vi "niRFUtil MEAS Estimate IQ Imbalances.vi"(8 "Reference Waveform":T2 {"y" format="%.2f"; "dx" format="%^.2e"; "x0" format="%^.2e"}, 10 "Measured Waveform":T2 {"y" format="%.2f"; "dx" format="%^.2e"; "x0" format="%^.2e"}) -> (0 "Phase Imbalance (rad)":sgl, 1 "Gain Imbalance g (lin)":sgl, 2 "Channel Phase Offset (rad)":sgl, 3 "Normalization Factor (lin)":sgl, 4 "Imbalance Matrix":T1)   [LabVIEW 2015, in "niRFUtil.lvlib"]
doc: "<b>Joint Estmator for IQ gain and phase imbalance and channel gain and phase</b>\n\nThe VI estimates the IQ gain and phase imbalances together with channel gain and phase. In presence of IQ imbalances, these parameters depend on each other and need a joint estimation. \n\nAssumptions:\n1. Arbitrary complex time-domain baseband signal and corresponding complex time-domain baseband reference signal\n2. Frequency offset free input signal\n3. Arbitrary gain scaling of input signal\n4. Origin Offset free input signal \n\nThe estimation algorithm is documented in \n//RfProtocols/Kraken/niCDMA2k/dev/2.0/group/NID_Documents/General/IqImbalanceEstimation/IqImbalanceEstimation.pdf \n\nThe model used for definition of gain and phase imbalance is taken from:\nA. Georgiadis, \"Gain, phase imbalance, and phase noise effects on error vector magnitude,\" in IEEE Transactions on Vehicular Technology, vol. 53, no. 2, pp. 443-449, March 2004."
uses:
  niRFUtil.lvlib
  Includes/niRFUtil INC Complex Waveform.ctl
  Includes/niRFUtil INC Complex Array.ctl
  <vilib>/Analysis/Matrix/Datatypes/RealMatrix.ctl
  <vilib>/Analysis/Matrix/Numeric/Conversions/Array To Matrix - RA2.vi
  <vilib>/Analysis/Matrix/NI_Matrix.lvlib
panel:
  out "phaseChannelRef":dbl
  out "phaseImbalanceRef":dbl
  out "Gain ImbalanceRef (log)":dbl
  out "ChannelGain":dbl
  out "Gain ImbalanceRef (lin)":dbl
  out "phaseChannelRefDeg":dbl
  out "phaseImbalanceRefDeg":dbl
  out "Gain Imbalance g (dB)":sgl
  out "Channel Phase Offset (deg)":sgl
  out "Phase Imbalance (deg)":sgl
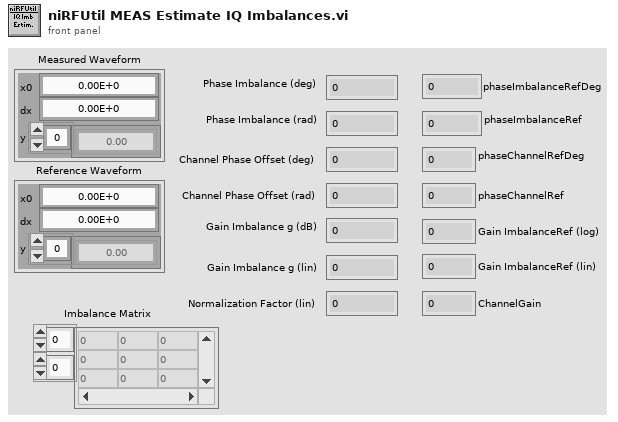
[diagram p1: front panel]
types:
  T1 = typedef "NI_Matrix.lvlib/RealMatrix.ctl" = dbl[][]
  T2 = typedef "niRFUtil.lvlib/niRFUtil INC Complex Waveform.ctl" = cluster{"x0":dbl, "dx":dbl, "y":T3}
  T3 = typedef "niRFUtil.lvlib/niRFUtil INC Complex Array.ctl" = csg[]
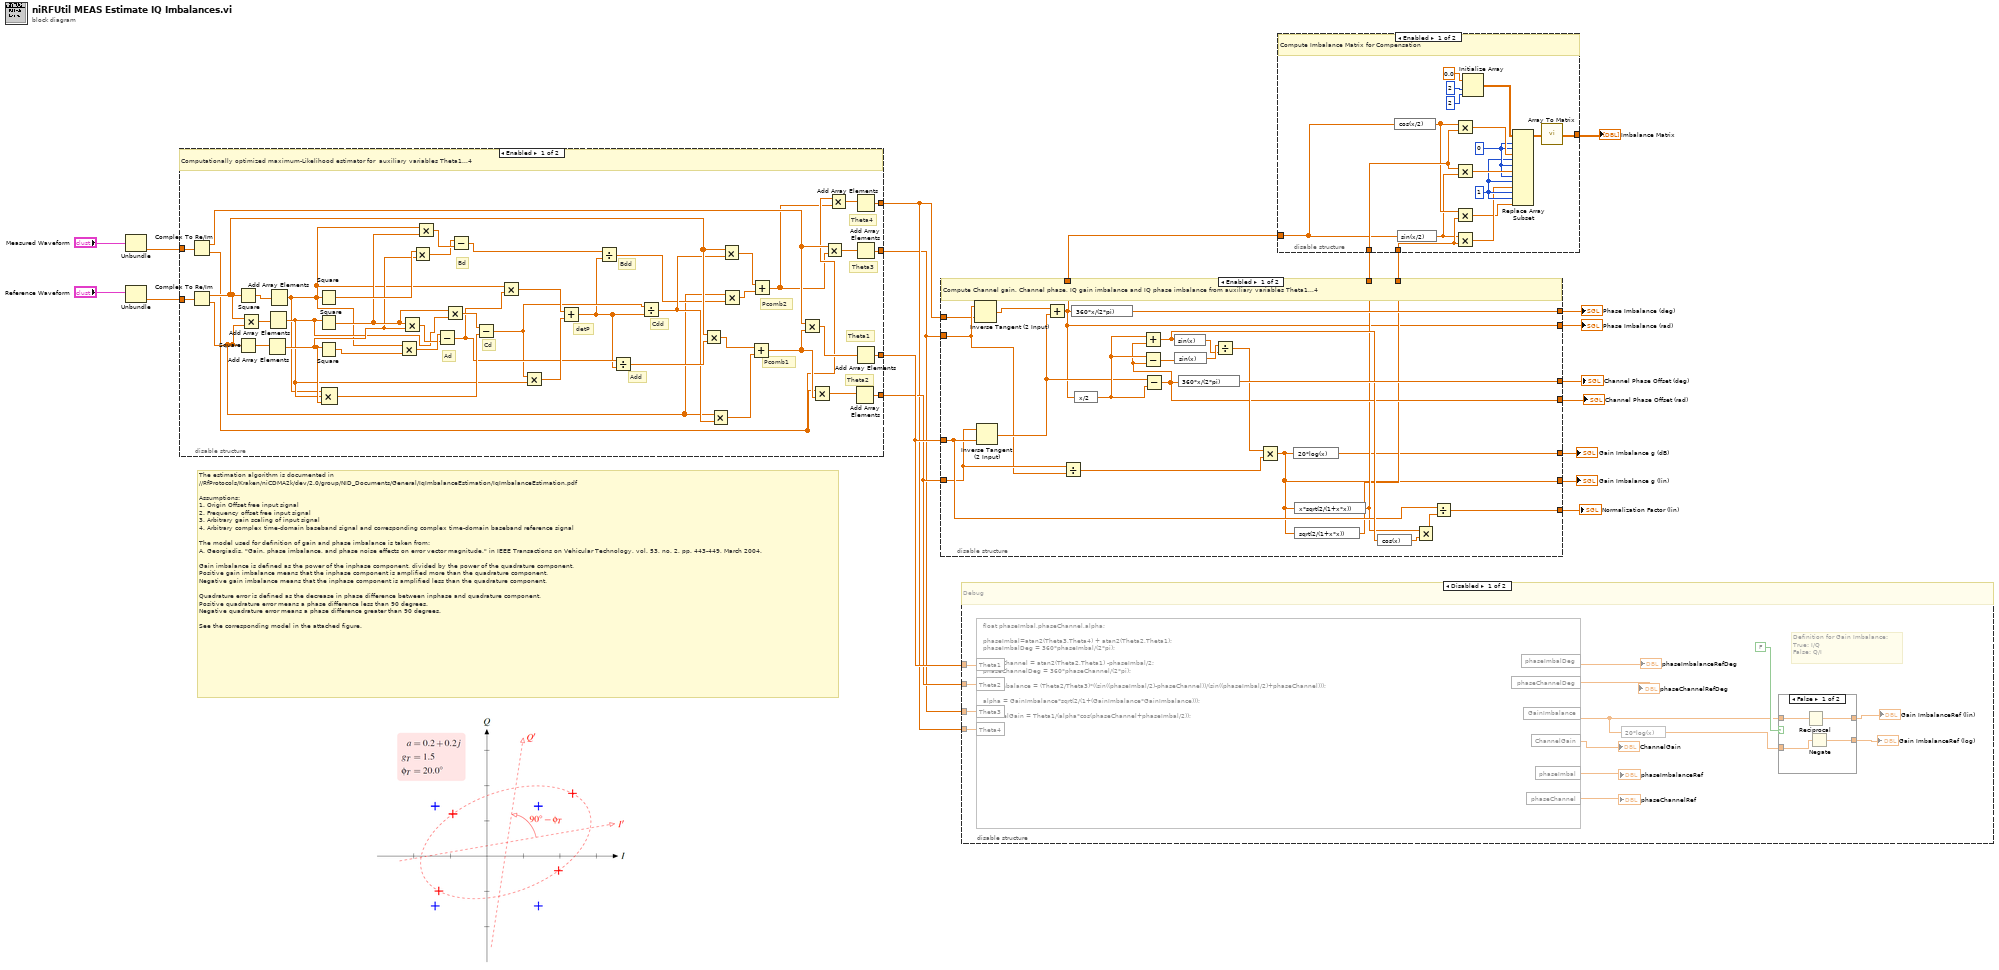
[diagram p0: block diagram]
diagram:
  # "The estimation algorithm is documented in \n//RfProtocols/Kraken/niCDMA2k/dev/2.0/group/NID_Documents/General/IqImbalanceEstimation/IqImbalanceEstimation.pdf \n\nAssumptions:\n1. Origin Offset free input signal\n2. Frequency offset free input signal\n3. Arbitrary gain scaling of input signal\n4. Arbitrary complex time-domain baseband signal and corresponding complex time-domain baseband reference signal\n\nThe model used for definition of gain and phase imbalance is taken from:\nA. Georgiadis, \"Gain, phase imbalance, and phase noise effects on error vector magnitude,\" in IEEE Transactions on Vehicular Technology, vol. 53, no. 2, pp. 443-449, March 2004.\n\nGain imbalance is defined as the power of the inphase component, divided by the power of the quadrature component.\nPositive gain imbalance means that the inphase component is amplified more than the quadrature component.\nNegative gain imbalance means that the inphase component is amplified less than the quadrature component.\n\nQuadrature error is defined as the decrease in phase difference between inphase and quadrature component. \nPositive quadrature error means a phase difference less than 90 degrees.\nNegative quadrature error means a phase difference greater than 90 degrees.\n\nSee the corresponding model in the attached figure."
  n1 = Unbundle("Measured Waveform") -> ("y"=w17:T3)  [unwired: 2 out]
  n2 = Unbundle("Reference Waveform") -> ("y"=w16:T3)  [unwired: 2 out]
  n3 = disable-structure shown="Enabled" {
    disable-tunnel: w17 -> [w63 _]
    disable-tunnel: w16 -> [w62 _]
    disable-tunnel: [w23 _] -> w12
    disable-tunnel: [w22 _] -> w11
    disable-tunnel: [w21 _] -> w1
    disable-tunnel: [w20 _] -> w10
    frame Enabled {
      # "Theta4"
      # "Theta3"
      # "Pcomb2"
      # "Pcomb1"
      # "Bdd"
      # "Theta2"
      # "Theta1"
      # "Cdd"
      # "Add"
      # "detP"
      # "Cd"
      # "Bd"
      # "Ad"
      # "Computationally optimized maximum-Likelihood estimator for  auxiliary variables Theta1...4"
      n4 = Complex To Re/Im(x + iy=w63) -> (x=w28:sgl[], y=w27:sgl[])
      n5 = Complex To Re/Im(x + iy=w62) -> (x=w32:sgl[], y=w29:sgl[])
      n6 = Square(x=w32) -> (x^2=w61:sgl[])
      n7 = Square(x=w29) -> (x^2=w59:sgl[])
      n8 = Multiply(x=w32, y=w29) -> (x*y=w60:sgl[])
      n9 = Add Array Elements(numeric array=w59) -> (sum=w51:sgl)
      n10 = Add Array Elements(numeric array=w60) -> (sum=w48:sgl)
      n11 = Add Array Elements(numeric array=w61) -> (sum=w47:sgl)
      n12 = Square(x=w47) -> (x^2=w53:sgl)
      n13 = Square(x=w48) -> (x^2=w52:sgl)
      n14 = Square(x=w51) -> (x^2=w58:sgl)
      n15 = Compound Arithmetic op=MULTIPLY(w47, w48, w51) -> (w49:sgl)
      n16 = Multiply(x=w47, y=w58) -> (x*y=w57:sgl)
      n17 = Multiply(x=w52, y=w51) -> (x*y=w56:sgl)
      n18 = Multiply(x=w53, y=w51) -> (x*y=w54:sgl)
      n19 = Multiply(x=w47, y=w52) -> (x*y=w55:sgl)
      n20 = Subtract(x=w57, y=w56) -> (x-y=w44:sgl)
      n21 = Multiply(x=w52, y=w48) -> (x*y=w50:sgl)
      n22 = Subtract(x=w54, y=w55) -> (x-y=w36:sgl)
      n23 = Subtract(x=w50, y=w49) -> (x-y=w43:sgl)
      n24 = Multiply(x=w47, y=w44) -> (x*y=w46:sgl)
      n25 = Multiply(x=w43, y=w48) -> (x*y=w45:sgl)
      n26 = Add(x=w46, y=w45) -> (x+y=w35:sgl)
      n27 = Divide(x=w36, y=w35) -> (x/y=w30:sgl)
      n28 = Divide(x=w44, y=w35) -> (x/y=w42:sgl)
      n29 = Divide(x=w43, y=w35) -> (x/y=w31:sgl)
      n30 = Multiply(x=w32, y=w42) -> (x*y=w41:sgl[])
      n31 = Multiply(x=w29, y=w31) -> (x*y=w40:sgl[])
      n32 = Multiply(x=w32, y=w31) -> (x*y=w33:sgl[])
      n33 = Multiply(x=w29, y=w30) -> (x*y=w34:sgl[])
      n34 = Add(x=w41, y=w40) -> (x+y=w39:sgl[])
      n35 = Add(x=w33, y=w34) -> (x+y=w26:sgl[])
      n36 = Multiply(x=w28, y=w39) -> (x*y=w38:sgl[])
      n37 = Multiply(x=w27, y=w39) -> (x*y=w37:sgl[])
      n38 = Multiply(x=w28, y=w26) -> (x*y=w24:sgl[])
      n39 = Multiply(x=w27, y=w26) -> (x*y=w25:sgl[])
      n40 = Add Array Elements(numeric array=w37) -> (sum=w22:sgl)
      n41 = Add Array Elements(numeric array=w25) -> (sum=w20:sgl)
      n42 = Add Array Elements(numeric array=w24) -> (sum=w21:sgl)
      n43 = Add Array Elements(numeric array=w38) -> (sum=w23:sgl)
    }
    frame Disabled {
    }
  }
  n44 = disable-structure shown="Enabled" {
    disable-tunnel: [w86 _] -> w15
    disable-tunnel: [w85 _] -> w14
    disable-tunnel: [w74 _] -> w13
    disable-tunnel: w12 -> [w73 _]
    disable-tunnel: w11 -> [w72 _]
    disable-tunnel: w1 -> [w71 _]
    disable-tunnel: w10 -> [w70 _]
    disable-tunnel: [w69 _] -> w9
    disable-tunnel: [w65 _] -> w8
    disable-tunnel: [w64 _] -> w7
    disable-tunnel: [w68 _] -> w6
    disable-tunnel: [w67 _] -> w5
    disable-tunnel: [w66 _] -> w3
    disable-tunnel: [w66 _] -> w2
    frame Enabled {
      # "Compute Channel gain, Channel phase, IQ gain imbalance and IQ phase imbalance from auxiliary variables Theta1...4"
      n45 = Inverse Tangent (2 Input)(1:w70, 2:w71) -> (0:w87:sgl)
      n46 = Inverse Tangent (2 Input)(1:w73, 2:w72) -> (0:w83:sgl)
      n47 = Add(x=w87, y=w83) -> (x+y=w66:sgl)
      n48 = Divide(x=w72, y=w71) -> (x/y=w79:sgl)
      n49 = expression code="360*x/(2*pi)"(w66) -> (w86:sgl)
      n50 = expression code="x/2"(w66) -> (w84:sgl)
      n51 = Subtract(x=w83, y=w84) -> (x-y=w69:sgl)
      n52 = Add(x=w84, y=w69) -> (x+y=w77:sgl)
      n53 = Subtract(x=w84, y=w69) -> (x-y=w82:sgl)
      n54 = expression code="sin(x)"(w77) -> (w80:sgl)
      n55 = expression code="sin(x)"(w82) -> (w81:sgl)
      n56 = expression code="360*x/(2*pi)"(w69) -> (w85:sgl)
      n57 = Divide(x=w81, y=w80) -> (x/y=w78:sgl)
      n58 = Multiply(x=w78, y=w79) -> (x*y=w64:sgl)
      n59 = expression code="20*log(x)"(w64) -> (w65:sgl)
      n60 = expression code="x*sqrt(2/(1+x*x))"(w64) -> (w68:sgl)
      n61 = expression code="sqrt(2/(1+x*x))"(w64) -> (w67:sgl)
      n62 = expression code="cos(x)"(w77) -> (w76:sgl)
      n63 = Multiply(x=w68, y=w76) -> (x*y=w75:sgl)
      n64 = Divide(x=w73, y=w75) -> (x/y=w74:sgl)
    }
    frame Disabled {
    }
  }
  "Phase Imbalance (deg)" <- w15
  "Channel Phase Offset (deg)" <- w14
  "Gain Imbalance g (dB)" <- w8
  "Gain Imbalance g (lin)" <- w7
  "Normalization Factor (lin)" <- w13
  "Channel Phase Offset (rad)" <- w9
  "Phase Imbalance (rad)" <- w3
  n65 = disable-structure shown="Disabled" {
    disable-tunnel: w12 -> [w101 _]
    disable-tunnel: w11 -> [w100 _]
    disable-tunnel: w1 -> [w99 _]
    disable-tunnel: w10 -> [w98 _]
    frame Disabled {
      # "Definition for Gain Imbalance:\nTrue: I/Q\nFalse: Q/I"
      # "Debug"
      n66 = formula code="float phaseImbal,phaseChannel,alpha;\n\nphaseImbal=atan2(Theta3,Theta4) + atan2(Theta2,Theta1);\nphaseImbalDeg = 360*phaseImbal/(2*pi);\n\nphaseChannel = atan2(Theta2,Theta1) -phaseImbal/2;\nphaseChannelDeg = 360*phaseChannel/(2*pi);\n\nGainImbalance = (Theta2/Theta3)*((sin((phaseImbal/2)-phaseChannel))/(sin((phaseImbal/2)+phaseChannel)));\n\nalpha = GainImbalance*sqrt(2/(1+(GainImbalance*GainImbalance)));\n\nChannelGain = Theta1/(alpha*cos(phaseChannel+phaseImbal/2));"("Theta1"=w101, "Theta2"=w100, "Theta3"=w99, "Theta4"=w98) -> ("phaseImbalDeg"=→"phaseImbalanceRefDeg":dbl, "phaseChannelDeg"=→"phaseChannelRefDeg":dbl, "GainImbalance"=w89:dbl, "ChannelGain"=→"ChannelGain":dbl, "phaseImbal"=→"phaseImbalanceRef":dbl, "phaseChannel"=→"phaseChannelRef":dbl)
      n67 = expression code="20*log(x)"(w89) -> (w91:dbl)
      n68 = case shown="False" FALSE {
        tunnel: [w105 w107] -> w92
        tunnel: w91 -> [w104 w107]
        tunnel: w89 -> [w103 w106]
        tunnel: [w102 w106] -> w88
        frame False {
          n69 = Reciprocal(x=w103) -> (1/x=w102:dbl)
          n70 = Negate(x=w104) -> (-x=w105:dbl)
        }
        frame True {
        }
      }
      "Gain ImbalanceRef (lin)" <- w88
      "Gain ImbalanceRef (log)" <- w92
    }
    frame Enabled {
    }
  }
  n71 = disable-structure shown="Enabled" {
    disable-tunnel: w6 -> [w124 _]
    disable-tunnel: w5 -> [w115 _]
    disable-tunnel: [w109 _] -> w4
    disable-tunnel: w2 -> [w108 _]
    frame Enabled {
      w116 = 1 ("index (row)")
      w117 = 0 ("index (row)")
      # "Compute Imbalance Matrix for Compensation"
      n72 = expression code="cos(x/2)"(w108) -> (w114:sgl)
      n73 = expression code="sin(x/2)"(w108) -> (w113:sgl)
      n74 = Multiply(x=w114, y=w124) -> (x*y=w119:sgl)
      n75 = Multiply(x=w124, y=w113) -> (x*y=w118:sgl)
      n76 = Multiply(x=w114, y=w115) -> (x*y=w111:sgl)
      n77 = Multiply(x=w113, y=w115) -> (x*y=w112:sgl)
      n78 = Initialize Array(0.0 ("element"), 2 ("dimension size"), 2 ("dimension size")) -> (w120:dbl[][])
      n79 = Replace Array Subset(array=w120, new element #1=w119, index (row) #1=w117, index (col) #1=w117, new element #2=w118, index (row) #2=w116, index (col) #2=w117, new element #3=w112, index (row) #3=w117, index (col) #3=w116, new element #4=w111, index (row) #4=w116, index (col) #4=w116) -> (w110:dbl[][])
      n80 = call-poly <vilib>:"Array To Matrix.vi"("Real 2D Array"=w110) -> ("Real Matrix"=w109:T1)
    }
    frame Disabled {
    }
  }
  "Imbalance Matrix" <- w4
